vi "Begin.vi"() -> (1 "CameraDevRef":T5)   [LabVIEW 2011]
doc: "Called before other user functions, this VI is expected to open initial I/O refnums, load in file data, and do all program initialization. Notice that the <B>error out</B> terminal is simply used for data flow. Wiring it to other structures or subVIs ensures that this VI runs first."
uses:
  <vilib>/Rock Robotics/WPI/Camera/WPI_CameraDevRef.ctl
  <vilib>/Rock Robotics/WPI/Encoder/WPI_EncoderDevRef.ctl
  <vilib>/Rock Robotics/SystemInterfaces/Encoder/FPGA_EncoderIdx.ctl
  <vilib>/Rock Robotics/SystemInterfaces/Counter/FPGA_CounterCtrSystemIndex.ctl
  <vilib>/Rock Robotics/WPI/Encoder/WPI_EncoderType.ctl
  <vilib>/Rock Robotics/WPI/Joystick/WPI_JoystickDeviceEnum.ctl
  <vilib>/Rock Robotics/SystemInterfaces/DIO/FPGA_DIOPWMChannel.ctl
  <vilib>/Rock Robotics/SystemInterfaces/Typedef/FPGA_TypedefDigitalModule.ctl
  <vilib>/Rock Robotics/WPI/MotorControl/WPI_MotorControlOpen Victor.vi
  Robot Global Data.vi
  <vilib>/Rock Robotics/SystemInterfaces/DIO/FPGA_DIORelayChannel.ctl
  <vilib>/Rock Robotics/WPI/Relay/WPI_RelayDirection.ctl
  <vilib>/Rock Robotics/SystemInterfaces/AI/FPGA_AIChannel.ctl
  <vilib>/Rock Robotics/WPI/Counter/WPI_CounterDigitalInputToDigitalSource.vi
  <vilib>/Rock Robotics/SystemInterfaces/DIO/FPGA_DIOChannel.ctl
  <vilib>/Rock Robotics/SystemInterfaces/AI/FPGA_AIGyroChannel.ctl
  <vilib>/Rock Robotics/WPI/MotorControl/WPI_MotorControlOpen Jaguar.vi
  <vilib>/Rock Robotics/SystemInterfaces/Typedef/FPGA_TypedefAnalogModule.ctl
  <vilib>/Utility/file.llb/Read From Spreadsheet File (DBL).vi
panel:
  out "LDriveEncoder 3":cluster{"status":bool}
  out "EncoderDevRef 3":T1={"DevStatus"={"status"=FALSE, "code"=0, "source"=""}, "EncoderIndex"=enum."Invalid", "CounterIndex"=enum."Invalid", "DistancePerCount"=1.0, "Decoding Type"=enum."4x"}
  out "EncoderDevRef 2":T1={"DevStatus"={"status"=FALSE, "code"=0, "source"=""}, "EncoderIndex"=enum."Invalid", "CounterIndex"=enum."Invalid", "DistancePerCount"=1.0, "Decoding Type"=enum."4x"}
  out "LDriveEncoder 2":errorcluster
  out "EncoderDevRef":T1={"DevStatus"={"status"=FALSE, "code"=0, "source"=""}, "EncoderIndex"=enum."Invalid", "CounterIndex"=enum."Invalid", "DistancePerCount"=1.0, "Decoding Type"=enum."4x"}
  out "LDriveEncoder":errorcluster
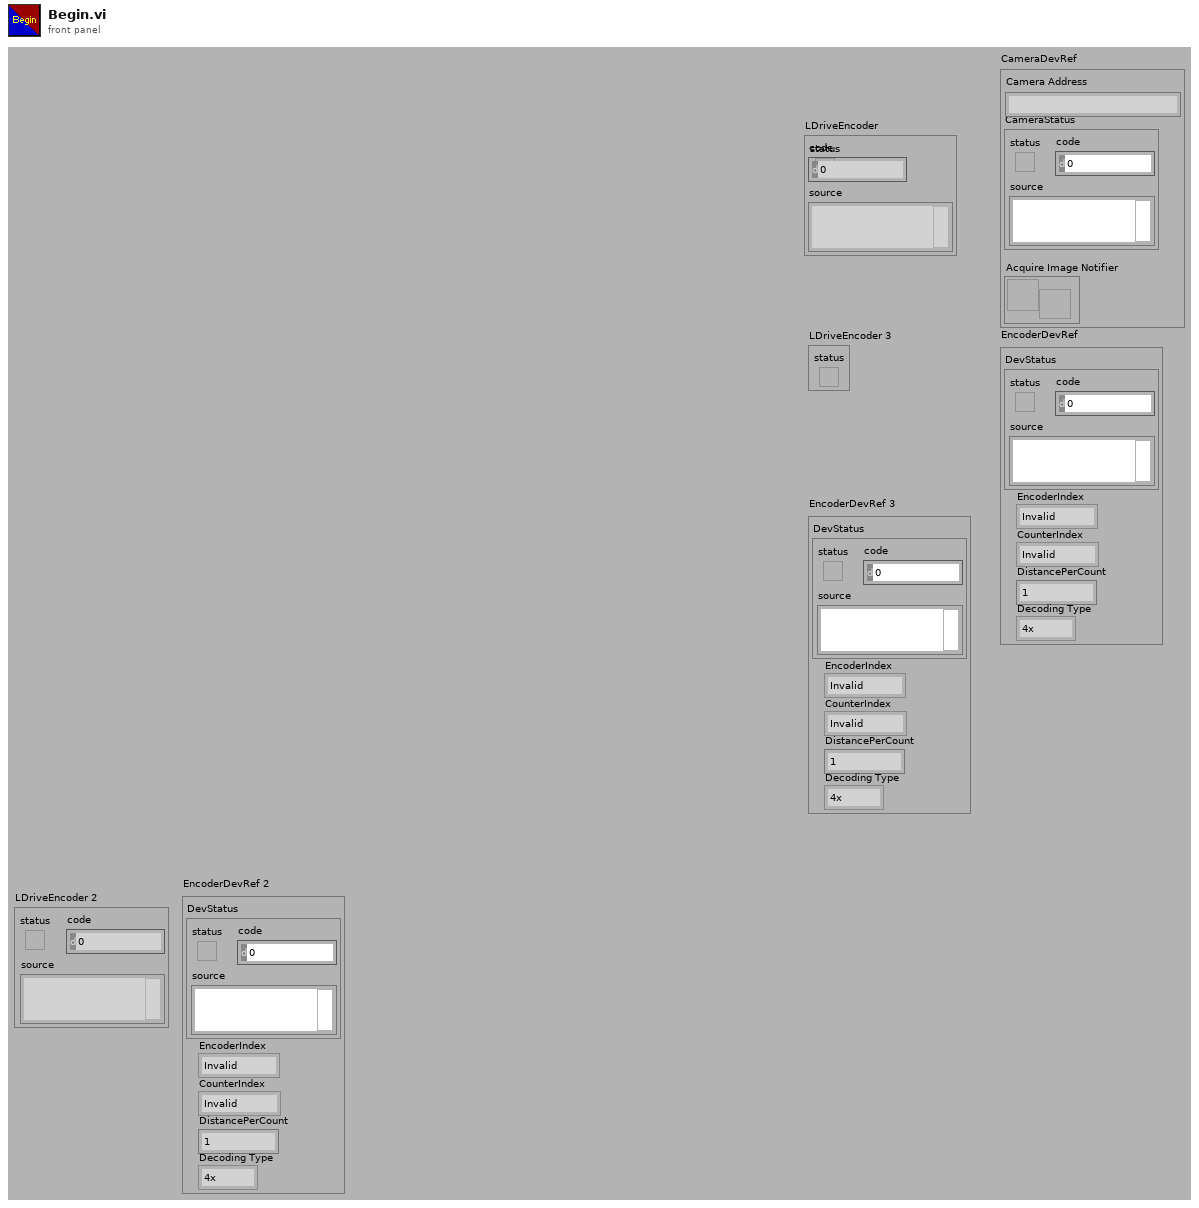
[diagram p1: front panel]
types:
  T1 = typedef "WPI_EncoderDevRef.ctl" = cluster{"DevStatus":errorcluster, "EncoderIndex":T2, "CounterIndex":T3, "DistancePerCount":dbl, "Decoding Type":T4}
  T2 = typedef "FPGA_EncoderIdx.ctl" = enum8{"Enc 0", "Enc 1", "Enc 2", "Enc 3", "Invalid"}
  T3 = typedef "FPGA_CounterCtrSystemIndex.ctl" = enum8{"Ctr 0", "Ctr 1", "Ctr 2", "Ctr 3", "Ctr 4", "Ctr 5", "Ctr 6", "Ctr 7", "Invalid"}
  T4 = typedef "WPI_EncoderType.ctl" = enum16{"1x", "2x", "4x"}
  T5 = typedef "WPI_CameraDevRef.ctl" = cluster{"Camera Address":string, "CameraStatus":errorcluster, "Acquire Image Notifier":refnum<notifier>}
  T6 = typedef "FPGA_TypedefDigitalModule.ctl" = enum16{"Digital Module 1", "Digital Module 2"}
  T7 = typedef "FPGA_DIOPWMChannel.ctl" = enum8{"PWM 1", "PWM 2", "PWM 3", "PWM 4", "PWM 5", "PWM 6", "PWM 7", "PWM 8", "PWM 9", "PWM 10", "Invalid"}
  T8 = typedef "WPI_JoystickDeviceEnum.ctl" = enum16{"USB 1", "USB 2", "USB 3", "USB 4", "Kinect 1", "Kinect 2"}
  T9 = typedef "FPGA_DIORelayChannel.ctl" = enum8{"Relay 1", "Relay 2", "Relay 3", "Relay 4", "Relay 5", "Relay 6", "Relay 7", "Relay 8", "Invalid"}
  T10 = typedef "FPGA_DIOChannel.ctl" = enum8{"DIO 1", "DIO 2", "DIO 3", "DIO 4", "DIO 5", "DIO 6", "DIO 7", "DIO 8", "DIO 9", "DIO 10", "DIO 11", "DIO 12", "DIO 13", "DIO 14", "Invalid"}
  T11 = typedef "WPI_MotorControlDeviceRef.ctl" = cluster{"DeviceStatus":errorcluster, "Type":enum16{"PWM", "CAN"}, "PWM":cluster{"Digital Module":T6, "PWM Channel":T7, "DeadBand":T12}, "CAN":cluster{"Device Number":u8, "Control Mode":T13, "Semaphore":T14, "Max Vout":dbl}, "Invert":bool, "TransformRef":T15, "InvTransformRef":T15}
  T12 = typedef "WPI_PWMDeadband.ctl" = cluster{"Name":string, "maxPositivePwm":i32, "minPositivePwm":i32, "centerPwm":i32, "maxNegativePwm":i32, "minNegativePwm":i32, "angularRange":u16}
  T13 = typedef "WPI_CANJaguar_ControlMode.ctl" = enum8{"Percent VBus", "Current", "Speed", "Position", "Voltage"}
  T14 = typedef "Semaphore RefNum" = refnum<k1>
  T15 = typedef "WPI_PWMTransform_ConPane.ctl" = refnum<vi>
  T16 = typedef "WPI_DigitalInputDevRef.ctl" = cluster{"DevStatus":errorcluster, "DIO Channel":T10, "Digital Module":T6}
  T17 = typedef "FPGA_CounterEncoderSourceConvertionLVSourceType.ctl" = cluster{"DevStatus":errorcluster, "AnalogTriggerMode?":bool, "DigitalMode":cluster{"Digital Module":T6, "DIO Channel":T18}, "AnalogTriggerMode":cluster{"AnalogTriggerIndex":T19, "OutputType":T20}}
  T18 = typedef "FPGA_DIODigitalSourceChannel.ctl" = enum8{"DIO 1", "DIO 2", "DIO 3", "DIO 4", "DIO 5", "DIO 6", "DIO 7", "DIO 8", "DIO 9", "DIO 10", "DIO 11", "DIO 12", "DIO 13", "DIO 14", "Disabled"}
  T19 = typedef "FPGA_AnalogTriggerIndex.ctl" = enum8{"Trig 0", "Trig 1", "Trig 2", "Trig 3", "Trig 4", "Trig 5", "Trig 6", "Trig 7", "Invalid"}
  T20 = typedef "FPGA_AnalogTriggerOutType.ctl" = enum16{"InWindow", "TriggerState", "Rising", "Falling"}
  T21 = typedef "WPI_RelayDevRef.ctl" = cluster{"DevStatus":errorcluster, "Relay Channel":T9, "Digital Module":T6, "Relay Direction":T22}
  T22 = typedef "WPI_RelayDirection.ctl" = enum16{"Both directions", "Forward only", "Reverse only"}
  T23 = typedef "FPGA_AIChannel.ctl" = enum8{"AI 1", "AI 2", "AI 3", "AI 4", "AI 5", "AI 6", "AI 7", "AI 8", "Invalid"}
  T24 = typedef "WPI_AnalogChannelDevRef.ctl" = cluster{"DevStatus":errorcluster, "Analog Module":T25, "Analog Channel":T23}
  T25 = typedef "FPGA_TypedefAnalogModule.ctl" = enum16{"Analog Module 1", "Analog Module 2"}
  T26 = typedef "WPI_CameraImageSize.ctl" = enum16{"640x480", "320x240", "160x120"}
  T27 = cluster{"fps":i32, "compression":i32, "Image Size":T26}
  T28 = typedef "WPI_CameraWhite Balance Values.ctl" = enum16{"Auto", "Fixed indoor", "Fixed outdoor 1", "Fixed outdoor 2", "Fixed fluorescent 1", "Fixed fluorescent 2", "Hold current"}
  T29 = typedef "WPI_CameraExposure Values.ctl" = enum16{"Auto", "Flicker-free 50 Hz", "Flicker-free 60 Hz", "Hold current"}
  T30 = typedef "WPI_ServoDeviceRef.ctl" = cluster{"DeviceStatus":errorcluster, "Digital Module":T6, "PWM Channel":T7, "DeadBand":T12}
  T31 = typedef "WPI_JoystickDevRef.ctl" = cluster{"Device":T8}
  T32 = typedef "FPGA_AIGyroChannel.ctl" = enum8{"AI 1", "AI 2", "Invalid"}
  T33 = typedef "WPI_GyroDevRef.ctl" = cluster{"DevStatus":errorcluster, "Analog Module":T25, "Analog Channel":T23, "Offset":dbl, "Gain (VoltsPerDegree/Second)":dbl}
  T34 = typedef "WPI_UltrasonicDeviceRef.ctl" = cluster{"DevStatus":errorcluster, "Ping Digital Module":T6, "Echo Digital Module":T6, "Ping Channel":T10, "Echo Channel":T10, "CntIndex":T3}
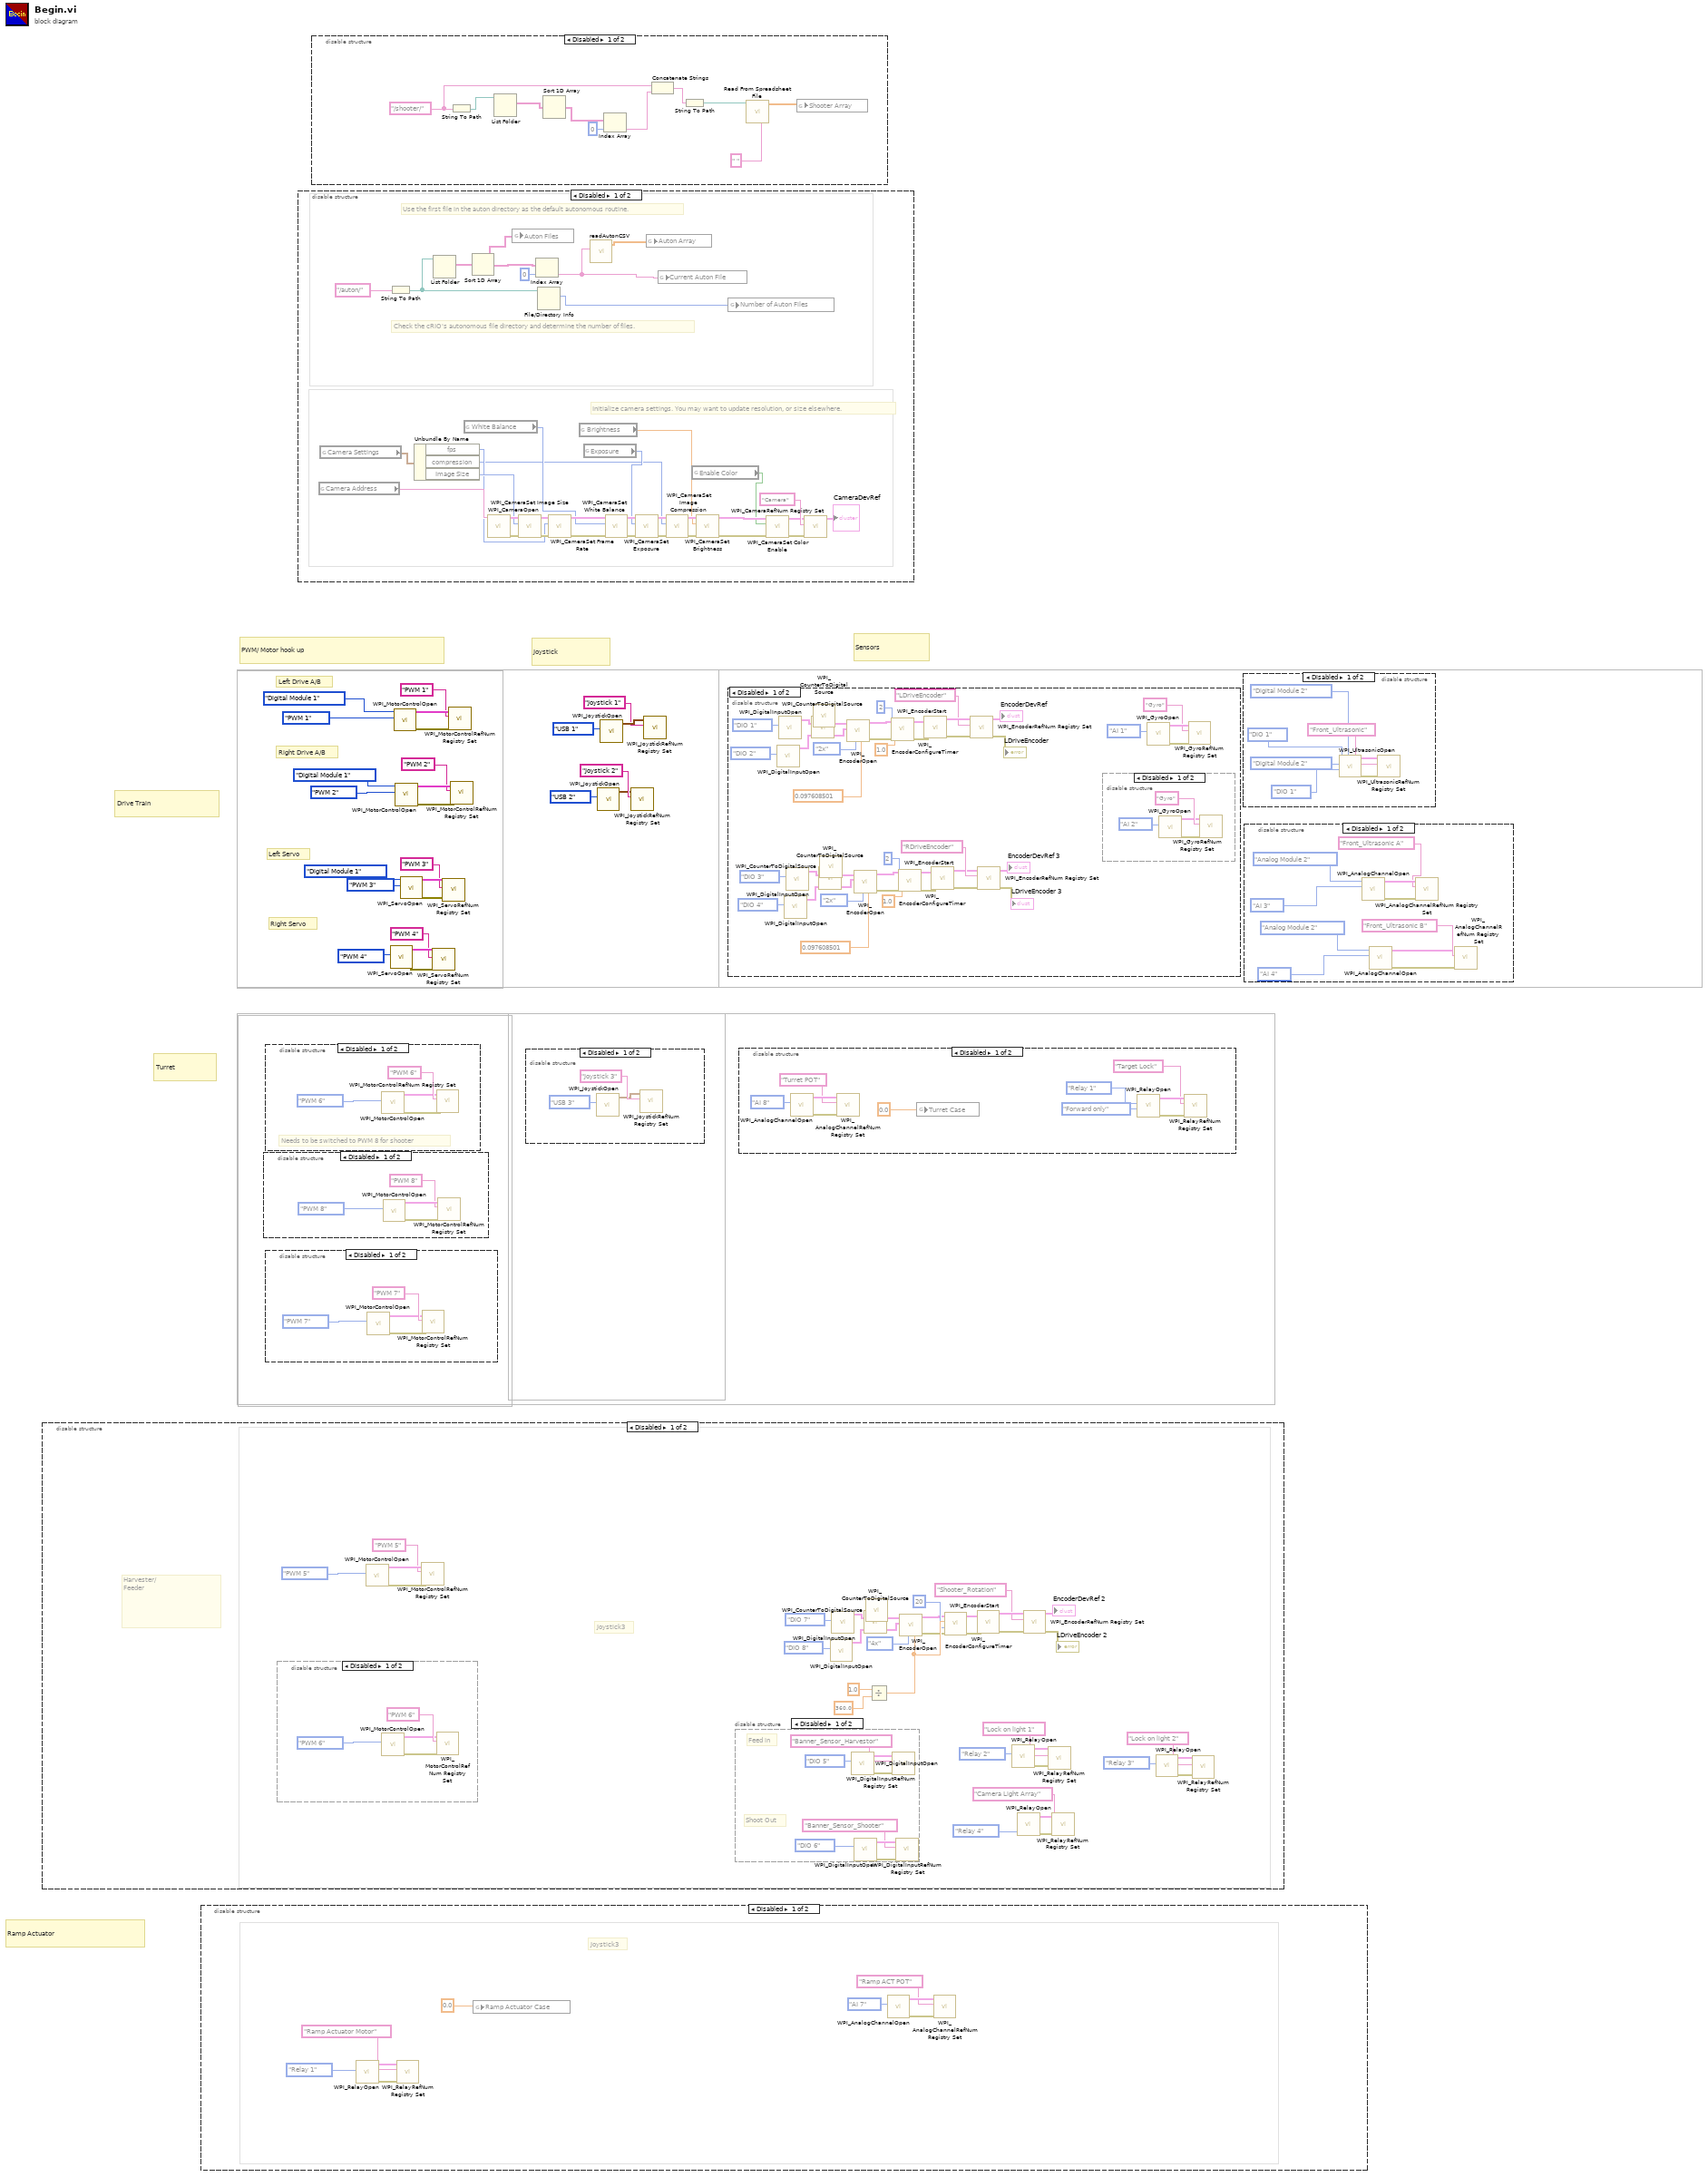
[diagram p0: block diagram]
diagram:
  # "Right Drive A/B"
  # "Left Drive A/B"
  # "Right Servo"
  # "Left Servo"
  # "Turret"
  # "Ramp Actuator"
  # "Drive Train"
  # "Sensors"
  # "Joystick"
  # "PWM/ Motor hook up"
  n1 = disable-structure shown="Disabled" {
    frame Disabled {
      # "Harvester/\nFeeder"
      # "Joystick3"
      n2 = disable-structure shown="Disabled" {
        frame Disabled {
          n3 = call-poly <vilib>:"WPI_MotorControlOpen.vi"("PWM Channel"=FPGA_DIOPWMChannel."PWM 6") -> ("error out"=w73:errorcluster, "MotorControlDeviceRef"=w71:T11)  [unwired: 9 in]
          n4 = call <vilib>:"WPI_MotorControlRefNum Registry Set.vi"("error in (no error)"=w73, "refnum name"="PWM 6", "MotorControlDevRef"=w71) -> ()  [unwired: 7 in, 2 out]
        }
        frame Enabled {
        }
      }
      n5 = call-poly <vilib>:"WPI_MotorControlOpen.vi"("PWM Channel"=FPGA_DIOPWMChannel."PWM 5") -> ("error out"=w58:errorcluster, "MotorControlDeviceRef"=w60:T11)  [unwired: 9 in]
      n6 = call <vilib>:"WPI_MotorControlRefNum Registry Set.vi"("error in (no error)"=w58, "refnum name"="PWM 5", "MotorControlDevRef"=w60) -> ()  [unwired: 7 in, 2 out]
      n7 = disable-structure shown="Disabled" {
        frame Disabled {
          # "Shoot Out"
          # "Feed in"
          n8 = call <vilib>:"WPI_DigitalInputOpen.vi"("DIO Channel"=FPGA_DIOChannel."DIO 5") -> ("error out"=w67:errorcluster, "DigitalInputDevRef"=w66:T16)  [unwired: 9 in]
          n9 = call <vilib>:"WPI_DigitalInputOpen.vi"("DIO Channel"=FPGA_DIOChannel."DIO 6") -> ("error out"=w64:errorcluster, "DigitalInputDevRef"=w63:T16)  [unwired: 9 in]
          n10 = call <vilib>:"WPI_DigitalInputRefNum Registry Set.vi"("error in (no error)"=w67, "refnum name"="Banner_Sensor_Harvestor", "DigitalInputDevRef"=w66) -> ()  [unwired: 7 in, 2 out]
          n11 = call <vilib>:"WPI_DigitalInputRefNum Registry Set.vi"("error in (no error)"=w64, "refnum name"="Banner_Sensor_Shooter", "DigitalInputDevRef"=w63) -> ()  [unwired: 7 in, 2 out]
        }
        frame Enabled {
        }
      }
      n12 = call <vilib>:"WPI_DigitalInputOpen.vi"("DIO Channel"=FPGA_DIOChannel."DIO 8") -> ("DigitalInputDevRef"=w42:T16)  [unwired: 9 in, 1 out]
      n13 = call <vilib>:"WPI_DigitalInputOpen.vi"("DIO Channel"=FPGA_DIOChannel."DIO 7") -> ("DigitalInputDevRef"=w39:T16)  [unwired: 9 in, 1 out]
      n14 = call-poly <vilib>:"WPI_CounterToDigitalSource.vi"("DigitalInputDevRef"=w42) -> ("Digital Source"=w43:T17)  [unwired: 6 in]
      n15 = call-poly <vilib>:"WPI_CounterToDigitalSource.vi"("DigitalInputDevRef"=w39) -> ("Digital Source"=w38:T17)  [unwired: 6 in]
      n16 = Divide(x=1.0, y=360.0) -> (x/y=w57:dbl)
      n17 = call <vilib>:"WPI_EncoderOpen.vi"("DistancePerCount"=w57, "Decoding Type"=WPI_EncoderType."4x", "BSource"=w43, "ASource"=w38) -> ("error out"=w46:errorcluster, "EncoderDevRef"=w47:T1)  [unwired: 6 in]
      n18 = call <vilib>:"WPI_EncoderConfigureTimer.vi"("error in (no error)"=w46, "Number Samples to Average"=u8 20, "Minimum Rate"=w57, "EncoderDevRef"=w47) -> ("error out"=w50:errorcluster, "EncoderDevRef"=w49:T1)  [unwired: 6 in]
      n19 = call <vilib>:"WPI_EncoderStart.vi"("error in (no error)"=w50, "EncoderDevRef"=w49) -> ("error out"=w52:errorcluster, "EncoderDevRef"=w51:T1)  [unwired: 8 in]
      n20 = call <vilib>:"WPI_RelayOpen.vi"("Relay Channel"=FPGA_DIORelayChannel."Relay 2") -> ("error out"=w35:errorcluster, "RelayDevRef"=w34:T21)  [unwired: 9 in]
      n21 = call <vilib>:"WPI_RelayOpen.vi"("Relay Channel"=FPGA_DIORelayChannel."Relay 4") -> ("error out"=w37:errorcluster, "RelayDevRef"=w36:T21)  [unwired: 9 in]
      n22 = call <vilib>:"WPI_EncoderRefNum Registry Set.vi"("error in (no error)"=w52, "refnum name"="Shooter_Rotation", "EncoderDevRef"=w51) -> ("error out"=→"LDriveEncoder 2":errorcluster, "EncoderDevRef"=→"EncoderDevRef 2":T1)  [unwired: 7 in]
      n23 = call <vilib>:"WPI_RelayRefNum Registry Set.vi"("error in (no error)"=w35, "refnum name"="Lock on light 1", "RelayDevRef"=w34) -> ()  [unwired: 7 in, 2 out]
      n24 = call <vilib>:"WPI_RelayRefNum Registry Set.vi"("error in (no error)"=w37, "refnum name"="Camera Light Array", "RelayDevRef"=w36) -> ()  [unwired: 7 in, 2 out]
      n25 = call <vilib>:"WPI_RelayOpen.vi"("Relay Channel"=FPGA_DIORelayChannel."Relay 3") -> ("error out"=w26:errorcluster, "RelayDevRef"=w27:T21)  [unwired: 9 in]
      n26 = call <vilib>:"WPI_RelayRefNum Registry Set.vi"("error in (no error)"=w26, "refnum name"="Lock on light 2", "RelayDevRef"=w27) -> ()  [unwired: 7 in, 2 out]
    }
    frame Enabled {
    }
  }
  n27 = disable-structure shown="Disabled" {
    frame Disabled {
      # "Joystick3"
      n28 = call <vilib>:"WPI_RelayOpen.vi"("Relay Channel"=FPGA_DIORelayChannel."Relay 1") -> ("error out"=w78:errorcluster, "RelayDevRef"=w77:T21)  [unwired: 9 in]
      n29 = call <vilib>:"WPI_RelayRefNum Registry Set.vi"("error in (no error)"=w78, "refnum name"="Ramp Actuator Motor", "RelayDevRef"=w77) -> ()  [unwired: 7 in, 2 out]
      n30 = global write "Robot Global Data.vi" "Ramp Actuator Case"(0.0 ("Ramp Actuator Case")) -> ()
      n31 = call <vilib>:"WPI_AnalogChannelOpen.vi"("Analog Channel"=FPGA_AIChannel."AI 7") -> ("error out"=w81:errorcluster, "AIDeviceRef"=w82:T24)  [unwired: 9 in]
      n32 = call <vilib>:"WPI_AnalogChannelRefNum Registry Set.vi"("error in (no error)"=w81, "refnum name"="Ramp ACT POT", "AIDeviceRef"=w82) -> ()  [unwired: 7 in, 2 out]
    }
    frame Enabled {
    }
  }
  n33 = disable-structure shown="Disabled" {
    frame Disabled {
      n34 = call-poly <vilib>:"WPI_MotorControlOpen.vi"("PWM Channel"=FPGA_DIOPWMChannel."PWM 8") -> ("error out"=w83:errorcluster, "MotorControlDeviceRef"=w85:T11)  [unwired: 9 in]
      n35 = call <vilib>:"WPI_MotorControlRefNum Registry Set.vi"("error in (no error)"=w83, "refnum name"="PWM 8", "MotorControlDevRef"=w85) -> ()  [unwired: 7 in, 2 out]
    }
    frame Enabled {
    }
  }
  n36 = disable-structure shown="Disabled" {
    frame Disabled {
      # "Needs to be switched to PWM 8 for shooter"
      n37 = call-poly <vilib>:"WPI_MotorControlOpen.vi"("PWM Channel"=FPGA_DIOPWMChannel."PWM 6") -> ("error out"=w90:errorcluster, "MotorControlDeviceRef"=w88:T11)  [unwired: 9 in]
      n38 = call <vilib>:"WPI_MotorControlRefNum Registry Set.vi"("error in (no error)"=w90, "refnum name"="PWM 6", "MotorControlDevRef"=w88) -> ()  [unwired: 7 in, 2 out]
    }
    frame Enabled {
    }
  }
  n39 = disable-structure shown="Disabled" {
    frame Disabled {
      n40 = call-poly <vilib>:"WPI_MotorControlOpen.vi"("PWM Channel"=FPGA_DIOPWMChannel."PWM 7") -> ("error out"=w94:errorcluster, "MotorControlDeviceRef"=w92:T11)  [unwired: 9 in]
      n41 = call <vilib>:"WPI_MotorControlRefNum Registry Set.vi"("error in (no error)"=w94, "refnum name"="PWM 7", "MotorControlDevRef"=w92) -> ()  [unwired: 7 in, 2 out]
    }
    frame Enabled {
    }
  }
  n42 = disable-structure shown="Disabled" {
    frame Disabled {
      # "Check the cRIO's autonomous file directory and determine the number of files."
      # "Use the first file in the auton directory as the default autonomous routine."
      # "Initialize camera settings. You may want to update resolution, or size elsewhere."
      n43 = global read "Robot Global Data.vi" "Camera Address"() -> (w116:string)
      n44 = global read "Robot Global Data.vi" "Camera Settings"() -> (w115:T27)
      n45 = String To Path(string="/auton/") -> (path=w101:path)
      n46 = Unbundle By Name(w115) -> ("fps"=w113:i32, "compression"=w110:i32, "Image Size"=w114:T26)
      n47 = List Folder(path=w101) -> (filenames=w100:string[])  [unwired: 1 in, 5 out]
      n48 = global read "Robot Global Data.vi" "White Balance"() -> (w112:T28)
      n49 = Sort 1D Array(array=w100) -> (sorted array=w95:string[])
      n50 = call <vilib>:"WPI_CameraOpen.vi"("Camera Address"=w116) -> ("error out"=w122:errorcluster, "CameraDevRef"=w123:T5)  [unwired: 1 in, 8 out]
      n51 = global write "Robot Global Data.vi" "Auton Files"(w95) -> ()
      n52 = call <vilib>:"WPI_CameraSet Image Size.vi"("error in (no error)"=w122, "Image Size"=w114, "CameraDevRef"=w123) -> ("error out"=w121:errorcluster, "CameraDevRef Out"=w124:T5)  [unwired: 7 out]
      n53 = Index Array(array=w95, index=0) -> (element=w97:string)
      n54 = File/Directory Info(path=w101) -> (size=w98:i64)  [unwired: 1 in, 6 out]
      n55 = call <vilib>:"WPI_CameraSet Frame Rate.vi"("error in (no error)"=w121, "Frame Rate (fps)"=w113, "CameraDevRef"=w124) -> ("error out"=w120:errorcluster, "CameraDevRef Out"=w126:T5)  [unwired: 7 out]
      n56 = global read "Robot Global Data.vi" "Brightness"() -> (w109:dbl)
      n57 = global read "Robot Global Data.vi" "Exposure"() -> (w111:T29)
      n58 = call "readAutonCSV.vi"("AutonFile"=w97) -> ("AutonArray"=w96:dbl[][])  [unwired: 7 in]
      n59 = call <vilib>:"WPI_CameraSet White Balance.vi"("error in (no error)"=w120, "White Balance"=w112, "CameraDevRef"=w126) -> ("error out"=w119:errorcluster, "CameraDevRef Out"=w125:T5)  [unwired: 7 out]
      n60 = call <vilib>:"WPI_CameraSet Exposure.vi"("error in (no error)"=w119, "Exposure"=w111, "CameraDevRef"=w125) -> ("error out"=w118:errorcluster, "CameraDevRef Out"=w128:T5)  [unwired: 7 out]
      n61 = global write "Robot Global Data.vi" "Auton Array"(w96) -> ()
      n62 = global write "Robot Global Data.vi" "Current Auton File"(w97) -> ()
      n63 = call <vilib>:"WPI_CameraSet Image Compression.vi"("error in (no error)"=w118, "Compression"=w110, "CameraDevRef"=w128) -> ("error out"=w117:errorcluster, "CameraDevRef Out"=w127:T5)  [unwired: 7 out]
      n64 = global read "Robot Global Data.vi" "Enable Color"() -> (w104:bool)
      n65 = call <vilib>:"WPI_CameraSet Brightness.vi"("error in (no error)"=w117, "Brightness"=w109, "CameraDevRef"=w127) -> ("error out"=w107:errorcluster, "CameraDevRef Out"=w108:T5)  [unwired: 7 out]
      n66 = global write "Robot Global Data.vi" "Number of Auton Files"(w98) -> ()
      n67 = call <vilib>:"WPI_CameraSet Color Enable.vi"("error in (no error)"=w107, "Color Enabled"=w104, "CameraDevRef"=w108) -> ("error out"=w105:errorcluster, "CameraDevRef Out"=w106:T5)  [unwired: 7 in]
      n68 = call <vilib>:"WPI_CameraRefNum Registry Set.vi"("error in (no error)"=w105, "refnum name"="Camera", "CameraDevRef"=w106) -> ("CameraDevRef"=→"CameraDevRef":T5)  [unwired: 8 out]
    }
    frame Enabled {
    }
  }
  n69 = disable-structure shown="Disabled" {
    frame Disabled {
      w138 = "/shooter/" ("string")
      n70 = String To Path(string=w138) -> (path=w139:path)
      n71 = List Folder(path=w139) -> (filenames=w137:string[])  [unwired: 1 in, 5 out]
      n72 = Sort 1D Array(array=w137) -> (sorted array=w136:string[])
      n73 = Index Array(array=w136, index=0) -> (element=w134:string)
      n74 = Concatenate Strings(w138, w134) -> (w133:string)
      n75 = String To Path(string=w133) -> (path=w132:path)
      n76 = call-poly <vilib>:"Read From Spreadsheet File.vi"("delimiter (\\t)"=" " ("delimiter (\\t)"), "file path (dialog if empty)"=w132) -> ("all rows"=w130:dbl[][])  [unwired: 5 in, 4 out]
      n77 = global write "Robot Global Data.vi" "Shooter Array"(w130) -> ()
    }
    frame Enabled {
    }
  }
  n78 = call <vilib>:"WPI_ServoOpen.vi"("PWM Channel"=FPGA_DIOPWMChannel."PWM 4") -> ("error out"=w1:errorcluster, "ServoDeviceRef"=w16:T30)  [unwired: 9 in]
  n79 = call-poly <vilib>:"WPI_MotorControlOpen.vi"("PWM Channel"=FPGA_DIOPWMChannel."PWM 1", "Digital Module (Module 1)"=FPGA_TypedefDigitalModule."Digital Module 1") -> ("error out"=w6:errorcluster, "MotorControlDeviceRef"=w9:T11)  [unwired: 8 in]
  n80 = call-poly <vilib>:"WPI_MotorControlOpen.vi"("PWM Channel"=FPGA_DIOPWMChannel."PWM 2", "Digital Module (Module 1)"=FPGA_TypedefDigitalModule."Digital Module 1") -> ("error out"=w7:errorcluster, "MotorControlDeviceRef"=w12:T11)  [unwired: 8 in]
  n81 = call <vilib>:"WPI_ServoOpen.vi"("PWM Channel"=FPGA_DIOPWMChannel."PWM 3", "Digital Module (Module 1)"=FPGA_TypedefDigitalModule."Digital Module 1") -> ("error out"=w2:errorcluster, "ServoDeviceRef"=w18:T30)  [unwired: 8 in]
  n82 = call <vilib>:"WPI_ServoRefNum Registry Set.vi"("error in (no error)"=w1, "refnum name"="PWM 4", "ServoDeviceRef"=w16) -> ()  [unwired: 7 in, 2 out]
  n83 = call <vilib>:"WPI_ServoRefNum Registry Set.vi"("error in (no error)"=w2, "refnum name"="PWM 3", "ServoDeviceRef"=w18) -> ()  [unwired: 7 in, 2 out]
  n84 = call <vilib>:"WPI_MotorControlRefNum Registry Set.vi"("error in (no error)"=w6, "refnum name"="PWM 1", "MotorControlDevRef"=w9) -> ()  [unwired: 7 in, 2 out]
  n85 = call <vilib>:"WPI_MotorControlRefNum Registry Set.vi"("error in (no error)"=w7, "refnum name"="PWM 2", "MotorControlDevRef"=w12) -> ()  [unwired: 7 in, 2 out]
  n86 = disable-structure shown="Disabled" {
    frame Disabled {
      n87 = call <vilib>:"WPI_JoystickOpen.vi"("JoystickDevice"=WPI_JoystickDeviceEnum."USB 3") -> ("JoystickDevRef"=w141:T31)  [unwired: 10 in]
      n88 = call <vilib>:"WPI_JoystickRefNum Registry Set.vi"("refnum name"="Joystick 3", "JoystickDevRef"=w141) -> ()  [unwired: 8 in, 2 out]
    }
    frame Enabled {
    }
  }
  n89 = call <vilib>:"WPI_JoystickOpen.vi"("JoystickDevice"=WPI_JoystickDeviceEnum."USB 2") -> ("JoystickDevRef"=w22:T31)  [unwired: 10 in]
  n90 = call <vilib>:"WPI_JoystickOpen.vi"("JoystickDevice"=WPI_JoystickDeviceEnum."USB 1") -> ("JoystickDevRef"=w25:T31)  [unwired: 10 in]
  n91 = call <vilib>:"WPI_JoystickRefNum Registry Set.vi"("refnum name"="Joystick 2", "JoystickDevRef"=w22) -> ()  [unwired: 8 in, 2 out]
  n92 = call <vilib>:"WPI_JoystickRefNum Registry Set.vi"("refnum name"="Joystick 1", "JoystickDevRef"=w25) -> ()  [unwired: 8 in, 2 out]
  n93 = disable-structure shown="Disabled" {
    frame Disabled {
      n94 = call <vilib>:"WPI_DigitalInputOpen.vi"("DIO Channel"=FPGA_DIOChannel."DIO 2") -> ("DigitalInputDevRef"=w166:T16)  [unwired: 9 in, 1 out]
      n95 = call <vilib>:"WPI_DigitalInputOpen.vi"("DIO Channel"=FPGA_DIOChannel."DIO 1") -> ("DigitalInputDevRef"=w163:T16)  [unwired: 9 in, 1 out]
      n96 = call <vilib>:"WPI_DigitalInputOpen.vi"("DIO Channel"=FPGA_DIOChannel."DIO 4") -> ("DigitalInputDevRef"=w157:T16)  [unwired: 9 in, 1 out]
      n97 = call <vilib>:"WPI_DigitalInputOpen.vi"("DIO Channel"=FPGA_DIOChannel."DIO 3") -> ("DigitalInputDevRef"=w160:T16)  [unwired: 9 in, 1 out]
      n98 = call-poly <vilib>:"WPI_CounterToDigitalSource.vi"("DigitalInputDevRef"=w166) -> ("Digital Source"=w167:T17)  [unwired: 6 in]
      n99 = call-poly <vilib>:"WPI_CounterToDigitalSource.vi"("DigitalInputDevRef"=w163) -> ("Digital Source"=w162:T17)  [unwired: 6 in]
      n100 = call-poly <vilib>:"WPI_CounterToDigitalSource.vi"("DigitalInputDevRef"=w157) -> ("Digital Source"=w156:T17)  [unwired: 6 in]
      n101 = call-poly <vilib>:"WPI_CounterToDigitalSource.vi"("DigitalInputDevRef"=w160) -> ("Digital Source"=w161:T17)  [unwired: 6 in]
      n102 = call <vilib>:"WPI_EncoderOpen.vi"("DistancePerCount"=0.097608501, "Decoding Type"=WPI_EncoderType."2x", "BSource"=w167, "ASource"=w162) -> ("error out"=w171:errorcluster, "EncoderDevRef"=w172:T1)  [unwired: 6 in]
      n103 = call <vilib>:"WPI_EncoderOpen.vi"("DistancePerCount"=0.097608501, "Decoding Type"=WPI_EncoderType."2x", "BSource"=w156, "ASource"=w161) -> ("error out"=w152:errorcluster, "EncoderDevRef"=w151:T1)  [unwired: 6 in]
      n104 = call <vilib>:"WPI_EncoderConfigureTimer.vi"("error in (no error)"=w171, "Number Samples to Average"=u8 2, "Minimum Rate"=1.0, "EncoderDevRef"=w172) -> ("error out"=w176:errorcluster, "EncoderDevRef"=w175:T1)  [unwired: 6 in]
      n105 = call <vilib>:"WPI_EncoderConfigureTimer.vi"("error in (no error)"=w152, "Number Samples to Average"=u8 2, "Minimum Rate"=1.0, "EncoderDevRef"=w151) -> ("error out"=w147:errorcluster, "EncoderDevRef"=w148:T1)  [unwired: 6 in]
      n106 = call <vilib>:"WPI_EncoderStart.vi"("error in (no error)"=w176, "EncoderDevRef"=w175) -> ("error out"=w178:errorcluster, "EncoderDevRef"=w177:T1)  [unwired: 8 in]
      n107 = call <vilib>:"WPI_EncoderStart.vi"("error in (no error)"=w147, "EncoderDevRef"=w148) -> ("error out"=w145:errorcluster, "EncoderDevRef"=w146:T1)  [unwired: 8 in]
      n108 = call <vilib>:"WPI_EncoderRefNum Registry Set.vi"("error in (no error)"=w178, "refnum name"="LDriveEncoder", "EncoderDevRef"=w177) -> ("error out"=→"LDriveEncoder":errorcluster, "EncoderDevRef"=→"EncoderDevRef":T1)  [unwired: 7 in]
      n109 = call <vilib>:"WPI_EncoderRefNum Registry Set.vi"("error in (no error)"=w145, "refnum name"="RDriveEncoder", "EncoderDevRef"=w146) -> ("error out"=→"LDriveEncoder 3":errorcluster, "EncoderDevRef"=→"EncoderDevRef 3":T1)  [unwired: 7 in]
      n110 = disable-structure shown="Disabled" {
        frame Disabled {
          n111 = call <vilib>:"WPI_GyroOpen.vi"("Analog Channel"=FPGA_AIGyroChannel."AI 2") -> ("error out"=w185:errorcluster, "GyroDevRef"=w186:T33)  [unwired: 8 in, 1 out]
          n112 = call <vilib>:"WPI_GyroRefNum Registry Set.vi"("error in (no error)"=w185, "refnum name"="Gyro", "GyroDevRef"=w186) -> ()  [unwired: 7 in, 2 out]
        }
        frame Enabled {
        }
      }
      n113 = call <vilib>:"WPI_GyroOpen.vi"("Analog Channel"=FPGA_AIGyroChannel."AI 1") -> ("error out"=w184:errorcluster, "GyroDevRef"=w183:T33)  [unwired: 8 in, 1 out]
      n114 = call <vilib>:"WPI_GyroRefNum Registry Set.vi"("error in (no error)"=w184, "refnum name"="Gyro", "GyroDevRef"=w183) -> ()  [unwired: 7 in, 2 out]
    }
    frame Enabled {
    }
  }
  n115 = disable-structure shown="Disabled" {
    frame Disabled {
      n116 = call <vilib>:"WPI_AnalogChannelOpen.vi"("Analog Channel"=FPGA_AIChannel."AI 8") -> ("error out"=w192:errorcluster, "AIDeviceRef"=w193:T24)  [unwired: 9 in]
      n117 = call <vilib>:"WPI_AnalogChannelRefNum Registry Set.vi"("error in (no error)"=w192, "refnum name"="Turret POT", "AIDeviceRef"=w193) -> ()  [unwired: 7 in, 2 out]
      n118 = global write "Robot Global Data.vi" "Turret Case"(0.0 ("Return To Home Case")) -> ()
      n119 = call <vilib>:"WPI_RelayOpen.vi"("Relay Direction"=WPI_RelayDirection."Forward only", "Relay Channel"=FPGA_DIORelayChannel."Relay 1") -> ("error out"=w197:errorcluster, "RelayDevRef"=w198:T21)  [unwired: 8 in]
      n120 = call <vilib>:"WPI_RelayRefNum Registry Set.vi"("error in (no error)"=w197, "refnum name"="Target Lock", "RelayDevRef"=w198) -> ()  [unwired: 7 in, 2 out]
    }
    frame Enabled {
    }
  }
  n121 = disable-structure shown="Disabled" {
    frame Disabled {
      n122 = call <vilib>:"WPI_UltrasonicOpen.vi"("Ping Digital Module (Module 1)"=FPGA_TypedefDigitalModule."Digital Module 2", "Echo DIO Channel"=FPGA_DIOChannel."DIO 1", "Echo Digital Module (Module 1)"=FPGA_TypedefDigitalModule."Digital Module 2", "Ping DIO Channel"=FPGA_DIOChannel."DIO 1") -> ("error out"=w205:errorcluster, "UltrasonicDevRef"=w204:T34)  [unwired: 6 in]
      n123 = call <vilib>:"WPI_UltrasonicRefNum Registry Set.vi"("error in (no error)"=w205, "refnum name"="Front_Ultrasonic", "UltrasonicDevRef"=w204) -> ()  [unwired: 7 in, 2 out]
    }
    frame Enabled {
    }
  }
  n124 = disable-structure shown="Disabled" {
    frame Disabled {
      n125 = call <vilib>:"WPI_AnalogChannelOpen.vi"("Analog Channel"=FPGA_AIChannel."AI 3", "Analog Module (Module 1)"=FPGA_TypedefAnalogModule."Analog Module 2") -> ("error out"=w211:errorcluster, "AIDeviceRef"=w210:T24)  [unwired: 8 in]
      n126 = call <vilib>:"WPI_AnalogChannelOpen.vi"("Analog Channel"=FPGA_AIChannel."AI 4", "Analog Module (Module 1)"=FPGA_TypedefAnalogModule."Analog Module 2") -> ("error out"=w206:errorcluster, "AIDeviceRef"=w207:T24)  [unwired: 8 in]
      n127 = call <vilib>:"WPI_AnalogChannelRefNum Registry Set.vi"("error in (no error)"=w211, "refnum name"="Front_Ultrasonic A", "AIDeviceRef"=w210) -> ()  [unwired: 7 in, 2 out]
      n128 = call <vilib>:"WPI_AnalogChannelRefNum Registry Set.vi"("error in (no error)"=w206, "refnum name"="Front_Ultrasonic B", "AIDeviceRef"=w207) -> ()  [unwired: 7 in, 2 out]
    }
    frame Enabled {
    }
  }
